vi "AM Modulation Demo (Baseband-Sine) - Mozart.vi"() -> ()   [LabVIEW 2013]
uses:
  <vilib>/sound2/lvsound2.llb/Sound File Info (path).vi
  <vilib>/sound2/lvsound2.llb/Sound File Read Open.vi
  <vilib>/sound2/lvsound2.llb/Sound File Read (DBL).vi
  <vilib>/Waveform/WDTOps.llb/WDT Get Waveform Subset DBL.vi
  <vilib>/express/express analysis/Spectral/Block/exnSpectralBlock spectral measurements power poly.vi
  <vilib>/express/express analysis/Spectral/Block/exnSpectralBlock spectral measurements power DDT.vi
  <vilib>/express/express analysis/Spectral/XNode/ExpressSpectralMeasurementsBlockNode.xnode
panel:
  out "After Rectifier 2":dynamicdata(graph)=[{"t0"=timestamp(0 s since 1904-01-01), "dt"=10.0, "Y"=array[50000 elements], "attributes"=variant("NI_ChannelName"=variant(string "Sine (Power Spectrum)"), "NI_ExpIsRelativeTime"=variant(bool TRUE), "NI_ExpStartTimeStamp"=variant(timestamp timestamp(3635665779.2842293 s since 1904-01-01)), "NI_ExpTimeStamp"=variant(timestamp timestamp(3635665779.2842293 s since 1904-01-01)), "NI_ExpXDimension"=variant(string "f"), "NI_OriginalChannelName"=variant(string "Sine"))}]
  in  "Path":path=path "D:/wendy/study/2023-2024Spring/EE206lab/lab/mozart.wav"
  in  "Duration":dbl=1000000.0 caption="Frequency"
  in  "WAV Sample Rate":dbl=44100.0 caption="dt"
  in  "Resample Rate":dbl=1000000.0 caption="Frequency"
  in  "LPF Cut-Off":dbl=10000.0 caption="Lower Cut-Off"
  in  "AWGN (dB)":dbl(slide)=0.6 caption="Standard deviation" scale=-20.0..50.0
  out "Recovered Signal":dynamicdata(graph)
  out "Baseband":dynamicdata(graph)
  out "AM Power Spectrum":dynamicdata(graph)
  out "AM Wave":dynamicdata(graph)
  in  "DC Offset":dbl=1.0
  in  "Carrier Amp.":dbl=1.0 caption="Amplitude"
  in  "stop":bool
  in  "Modulation Index":dbl(slide)=1.0 scale=0.0..5.0
  in  "Carrier Freq.":dbl=100000.0 caption="Frequency"
  out "After Rectifier":dynamicdata(graph)=[{"t0"=timestamp(0 s since 1904-01-01), "dt"=10.0, "Y"=array[50000 elements], "attributes"=variant("NI_ChannelName"=variant(string "Sine (Power Spectrum)"), "NI_ExpIsRelativeTime"=variant(bool TRUE), "NI_ExpStartTimeStamp"=variant(timestamp timestamp(3635665779.2842293 s since 1904-01-01)), "NI_ExpTimeStamp"=variant(timestamp timestamp(3635665779.2842293 s since 1904-01-01)), "NI_ExpXDimension"=variant(string "f"), "NI_OriginalChannelName"=variant(string "Sine"))}]
  # "Amplitude Modulation"
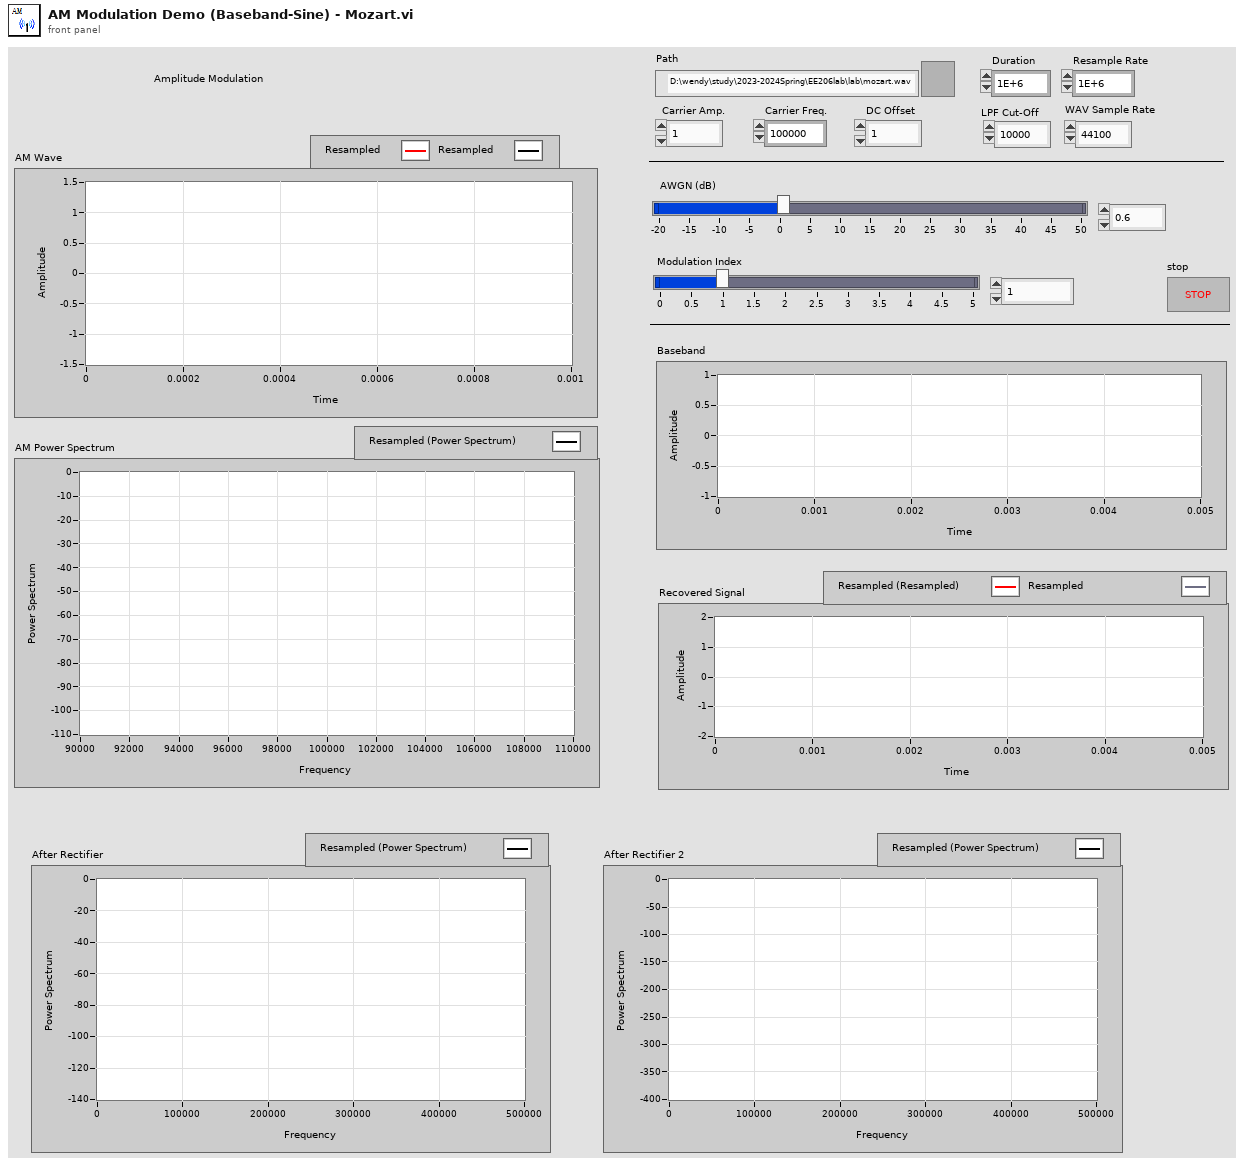
[diagram p1: front panel]
types:
  T1 = typedef "Sound File Refnum.ctl" = refnum<file>
  T2 = cluster{"averaging mode":u16, "weighting mode":u16, "number of averages":u32}
  T3 = cluster{"dB On (F)":bool, "unwrap phase (F)":bool, "convert to degree (F)":bool}
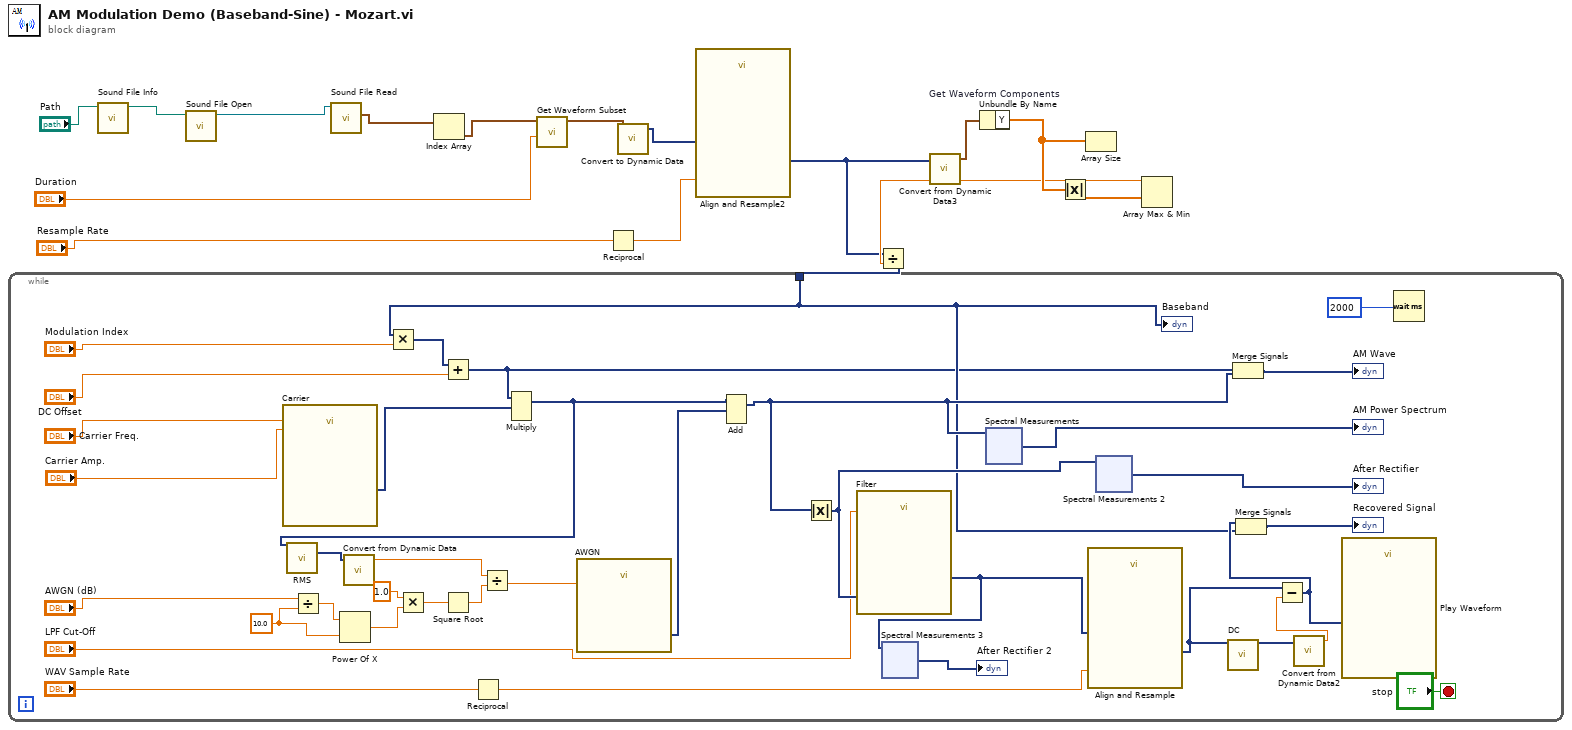
[diagram p0: block diagram]
diagram:
  n1 = call-poly <vilib>:"Sound File Info.vi"("path"="Path") -> ("path out"=w5:path)  [unwired: 7 in, 3 out]
  n2 = call-poly <vilib>:"Sound File Open.vi"("path"=w5) -> ("sound file refnum"=w15:T1)  [unwired: 9 in, 1 out]
  n3 = call-poly <vilib>:"Sound File Read.vi"("sound file refnum"=w15) -> ("data"=w14:waveform(dbl)[])  [unwired: 6 in, 4 out]
  n4 = Index Array "Index Array"(array=w14) -> (element=w13:waveform(dbl))  [unwired: 1 in]
  n5 = call-poly <vilib>:"Get Waveform Subset.vi"("duration"="Duration", "waveform in"=w13) -> ("waveform out"=w7:waveform(dbl))  [unwired: 4 in, 3 out]
  n6 = Reciprocal(x="Resample Rate") -> (1/x=w8:dbl)
  n7 = call "Convert to Dynamic Data"("Waveform"=w7) -> ("Dynamic Data Type"=w12:dynamicdata)  [unwired: 3 in]
  n8 = call "Align and Resample2"("dt"=w8, "Signals"=w12) -> ("Resampled Signals"=w2:dynamicdata)  [unwired: 7 in, 2 out]
  n9 = call "Convert from Dynamic Data3"("Dynamic Data Type"=w2) -> ("Waveform"=w1:waveform(dbl))  [unwired: 3 in]
  n10 = Unbundle By Name "Get Waveform Components"(w1) -> ("Y"=w11:dbl[])
  n11 = Absolute Value(x=w11) -> (abs(x)=w10:dbl[])
  n12 = Array Size(array=w11) -> ()  [unwired: 1 out]
  n13 = Array Max & Min(array=w10) -> (max value=w9:dbl)  [unwired: 3 out]
  n14 = Divide(x=w2, y=w9) -> (x/y=w6:dynamicdata)
  n15 = while {
    tunnel: w6 -> [w22]
    stop <- "stop" stop-if-true
    w36 = 10.0
    n16 = call "Carrier"("Frequency"="Carrier Freq.", "Amplitude"="Carrier Amp.") -> ("Sine"=w21:dynamicdata)  [unwired: 12 in, 1 out]
    n17 = Divide(x="AWGN (dB)", y=w36) -> (x/y=w43:dbl)
    n18 = Power Of X(1:w36, 2:w43) -> (0:w41:dbl)
    n19 = Multiply(x=w22, y="Modulation Index") -> (x*y=w51:dynamicdata)
    n20 = Multiply(x=1.0, y=w41) -> (x*y=w39:dbl)
    n21 = Add(x=w51, y="DC Offset") -> (x+y=w19:dynamicdata)
    n22 = Square Root(x=w39) -> (sqrt(x)=w38:dbl)
    n23 = Reciprocal(x="WAV Sample Rate") -> (1/x=w24:dbl)
    n24 = Multiply(1:w21, 2:w19) -> (0:w20:dynamicdata)  [unwired: 1 in, 1 out]
    n25 = call "RMS"("Signals"=w20) -> ("RMS"=w40:dynamicdata)  [unwired: 13 in, 1 out]
    n26 = call "Convert from Dynamic Data"("Dynamic Data Type"=w40) -> ("Scalar"=w37:dbl)  [unwired: 3 in]
    n27 = Divide(x=w37, y=w38) -> (x/y=w34:dbl)
    n28 = call "AWGN"("Standard deviation"=w34) -> ("DC with Gaussian Noise"=w35:dynamicdata)  [unwired: 13 in, 1 out]
    n29 = Add(1:w35, 2:w20) -> (0:w33:dynamicdata)  [unwired: 1 in, 1 out]
    n30 = Absolute Value(x=w33) -> (abs(x)=w32:dynamicdata)
    n31 = call "Filter"("Lower Cut-Off"="LPF Cut-Off", "Signal"=w32) -> ("Filtered Signal"=w18:dynamicdata)  [unwired: 8 in, 1 out]
    n32 = xnode "Spectral Measurements 3"("Signals"=w18) -> ("Power Spectrum"=→"After Rectifier 2":dynamicdata)  [unwired: 1 in, 1 out]
    n33 = xnode "Spectral Measurements"("Signals"=w33) -> ("Power Spectrum"=→"AM Power Spectrum":dynamicdata)  [unwired: 1 in, 1 out]
    n34 = call "Align and Resample"("dt"=w24, "Signals"=w18) -> ("Resampled Signals"=w28:dynamicdata)  [unwired: 7 in, 2 out]
    n35 = xnode "Spectral Measurements 2"("Signals"=w32) -> ("Power Spectrum"=→"After Rectifier":dynamicdata)  [unwired: 1 in, 1 out]
    n36 = call "DC"("Signals"=w28) -> ("Mean (DC)"=w26:dynamicdata)  [unwired: 13 in, 1 out]
    n37 = Merge Signals(w19, w33) -> (→"AM Wave":dynamicdata)
    n38 = call "Convert from Dynamic Data2"("Dynamic Data Type"=w26) -> ("Scalar"=w27:dbl)  [unwired: 3 in]
    n39 = Subtract(x=w28, y=w27) -> (x-y=w23:dynamicdata)
    n40 = Merge Signals(w23, w22) -> (→"Recovered Signal":dynamicdata)
    n41 = call "Play Waveform"("Data"=w23) -> ()  [unwired: 18 in, 1 out]
    n42 = Wait (ms)(milliseconds to wait=2000) -> ()  [unwired: 1 out]
    "Baseband" <- w22
  }
